vi "Store Static VI References for Subpanel.vi"(8 "error in (no error)":errorcluster, 11 "Step Configuration in":refnum<class "Step Configuration.lvclass">) -> (0 "error out":errorcluster, 3 "Step Configuration out":refnum<class "Step Configuration.lvclass">)   [LabVIEW 2026, in "Measurement Actor.lvlib" / "Step Configuration.lvclass"]
uses:
  Step Configuration.lvclass
  C:/Users/E2013170/Documents/GitHub/Measurement-Utility-Reference/source/configuration/Configuration.lvclass
  Logging Settings.vi
  configuration/Configuration.lvclass
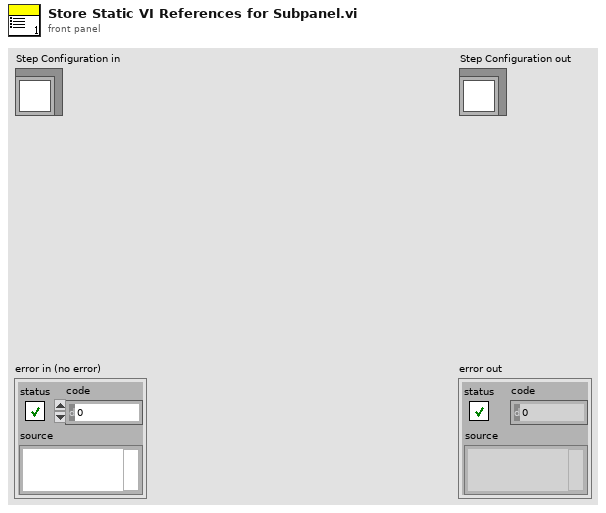
[diagram p1: front panel]
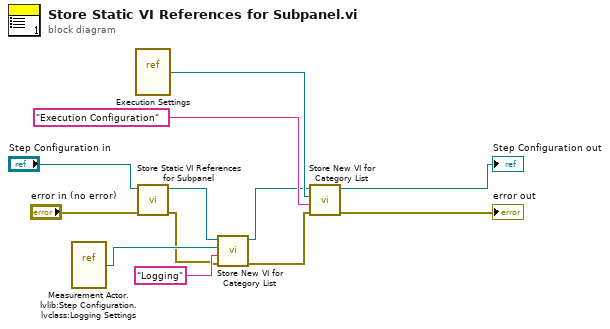
[diagram p0: block diagram]
diagram:
  n1 = vi-ref "Measurement Actor.lvlib:Step Configuration.lvclass:Logging Settings.vi"() -> (w6:refnum<vi>)
  n2 = vi-ref "Execution Settings.vi"() -> (w9:refnum<vi>)
  n3 = call-parent "Store Static VI References for Subpanel.vi"("error in (no error)"="error in (no error)", "Configuration in"="Step Configuration in") -> ("error out"=w2:errorcluster, "Configuration out"=w4:refnum<class "Step Configuration.lvclass">)  [unwired: 8 in]
  n4 = call "Store New VI for Category List.vi"("error in (no error)"=w2, "String"="Logging", "VI Refnum"=w6, "Configuration in"=w4) -> ("error out"=w1:errorcluster, "Configuration out"=w3:refnum<class "Step Configuration.lvclass">)  [unwired: 6 in]
  n5 = call "Store New VI for Category List.vi"("error in (no error)"=w1, "String"="Execution Configuration", "VI Refnum"=w9, "Configuration in"=w3) -> ("error out"=→"error out":errorcluster, "Configuration out"=→"Step Configuration out":refnum<class "Step Configuration.lvclass">)  [unwired: 6 in]
